vi "Init Data.vi"(10 "Data":T1) -> (3 "Msg out":refnum<class "Msg.lvclass">)   [LabVIEW 2020, in "Service.lvlib" / "Msg.lvclass"]
uses:
  Msg.lvclass
  Msg.lvclass/Msg.ctl
  Data.ctl
  Service.lvlib
  ServiceType/Enumeration.ctl
  ServiceType/ServiceType.lvlib
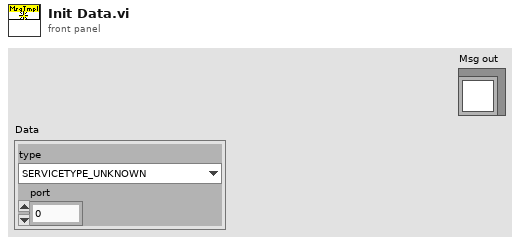
[diagram p1: front panel]
types:
  T1 = typedef "Service.lvlib/Data.ctl" = cluster{"type":T2, "port":i32}
  T2 = typedef "ServiceType.lvlib/Enumeration.ctl" = enum16{"SERVICETYPE_UNKNOWN", "SERVICETYPE_TCPSERVER", "SERVICETYPE_HTTPSERVER"}
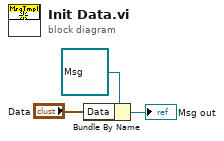
[diagram p0: block diagram]
diagram:
  n1 = Bundle By Name(cluster=refnum<class "Msg.lvclass"> refnum ("Msg out"), "Data"="Data") -> (→"Msg out":refnum<class "Msg.lvclass">)
